vi "FlushAutoModeQueue.vi"(8 "error in (no error)":errorcluster, 11 "Queue in":refnum<queue>) -> (0 "error out":errorcluster, 3 "Queue out":refnum<queue>)   [LabVIEW 2019, in "AutoMode.lvlib"]
uses:
  AutoMode.lvlib
  Cluster - AutoModeMessage.ctl
  Enum - AutoModeState.ctl
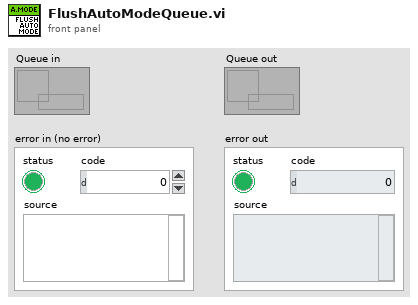
[diagram p1: front panel]
types:
  T1 = typedef "AutoMode.lvlib/Cluster - AutoModeMessage.ctl" = cluster{"Message":T2, "Data":variant}
  T2 = typedef "AutoMode.lvlib/Enum - AutoModeState.ctl" = enum16{"Initialize", "Idle", "UpdateConfig", "UpdateHWConfig", "BroadcastSettings", "Start", "CheckValidReportPath", "Winding", "WaitForWinding", "Unwind", "WaitForUnwind", "Stop", "Abort", "WriteDataToFile", "EventTriggered", "GenerateFilePath", "ZeroPosition", "GotoZero", "Error", "Exit"}
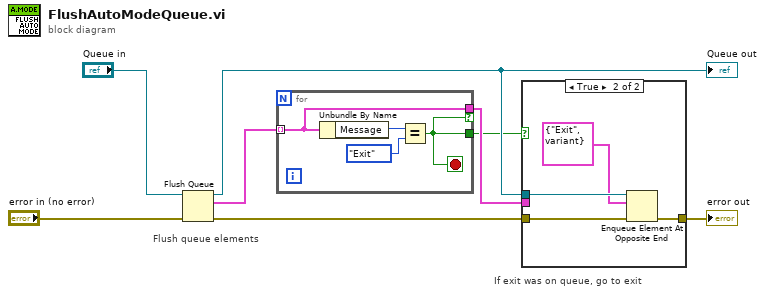
[diagram p0: block diagram]
diagram:
  # "If exit was on queue, go to exit"
  # "Flush queue elements"
  n1 = Flush Queue(queue="Queue in", error in (no error)="error in (no error)") -> (queue out=w3:refnum<queue>, remaining elements=w5:T1[], error out=w7:errorcluster)
  "Queue out" <- w3
  n2 = for {
    tunnel: w5 -> [w10] mode=indexing
    tunnel: [w9] -> w1
    tunnel: [w10] -> w2 if=w9
    stop <- w9 stop-if-true
    n3 = Unbundle By Name(w10) -> ("Message"=w12:T2)
    n4 = Equal?(x=w12, y=Enum_-_AutoModeState."Exit") -> (x = y?=w9:bool)
  }
  n5 = case shown="True" w1 {
    tunnel: w7 -> [w13 w17]
    tunnel: [w13 w16] -> w4
    tunnel: w3 -> [_ w15]
    tunnel: w2 -> [_ _]
    frame False {
    }
    frame True {
      n6 = Enqueue Element At Opposite End(queue=w15, element=T1 {"Message"=enum."Exit", "Data"=variant}, error in (no error)=w17) -> (error out=w16:errorcluster)  [unwired: 1 in, 2 out]
    }
  }
  "error out" <- w4
